vi "GV trigger delay.vi"() -> ()   [LabVIEW 2017]
panel:
  out "TriggerDelay_tick":u16
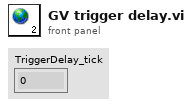
[diagram p1: front panel]
diagram:
